vi "Current Date & Time String (High Precision).vi"(8 "Error In":errorcluster) -> (0 "Error Out":errorcluster, 1 "on <Date> at <Time>":string, 2 "time string":string, 3 "date string":string)   [LabVIEW 2021]
doc: "<B>Error In</B> is passed unchanged to <B>Error Out</B> and is ignored"
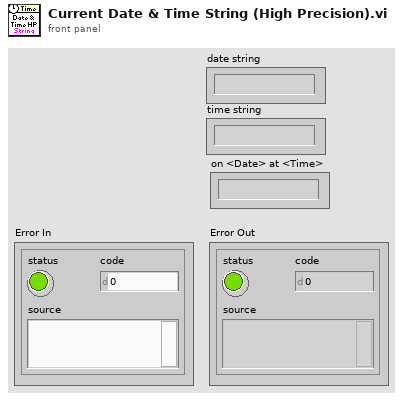
[diagram p1: front panel]
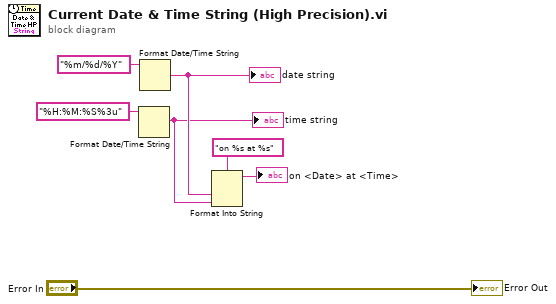
[diagram p0: block diagram]
diagram:
  n1 = Format Date/Time String(time format string (%c)="%H:%M:%S%3u") -> (date/time string=w2:string)  [unwired: 2 in]
  "time string" <- w2
  n2 = Format Date/Time String(time format string (%c)="%m/%d/%Y") -> (date/time string=w3:string)  [unwired: 2 in]
  "date string" <- w3
  n3 = Format Into String(format string="on %s at %s", w3, w2) -> (resulting string=→"on <Date> at <Time>":string)  [unwired: 2 in, 1 out]
  "Error Out" <- "Error In"
